vi "UpdateChannelWithParams.vi"(8 "error in":errorcluster, 10 "ParamArray":T1[](array[typedef]), 11 "channels in":T5 {"speed" items=["OWL429_HIGH_SPEED_CHANNEL", "OWL429_LOW_SPEED_CHANNEL"]; "Labels"."scheduleBuildUnit" items=["Millisecond", "Microsecond"]}) -> (0 "error out":errorcluster, 3 "channels out":T5 {"speed" items=["OWL429_HIGH_SPEED_CHANNEL", "OWL429_LOW_SPEED_CHANNEL"]; "Labels"."scheduleBuildUnit" items=["Millisecond", "Microsecond"]})   [LabVIEW 2016]
uses:
  Ballard Arinc-429 System Explorer.lvlib
  Controls/ARINCParam.ctl
  Controls/AIT_Label.ctl
  Controls/AIT_Channel.ctl
  Controls/AIT_Channel Array.ctl
  Controls/LabelInfo.ctl
  Controls/LabelParam.ctl
  Controls/ChannelParams.ctl
  Controls/AIT_Word.ctl
  Shared/Controls and Global/TransferType.ctl
  Shared/Ballard Arinc-429 Shared.lvlib
  Controls/Channel_direction.ctl
  Controls/Channel Speed.ctl
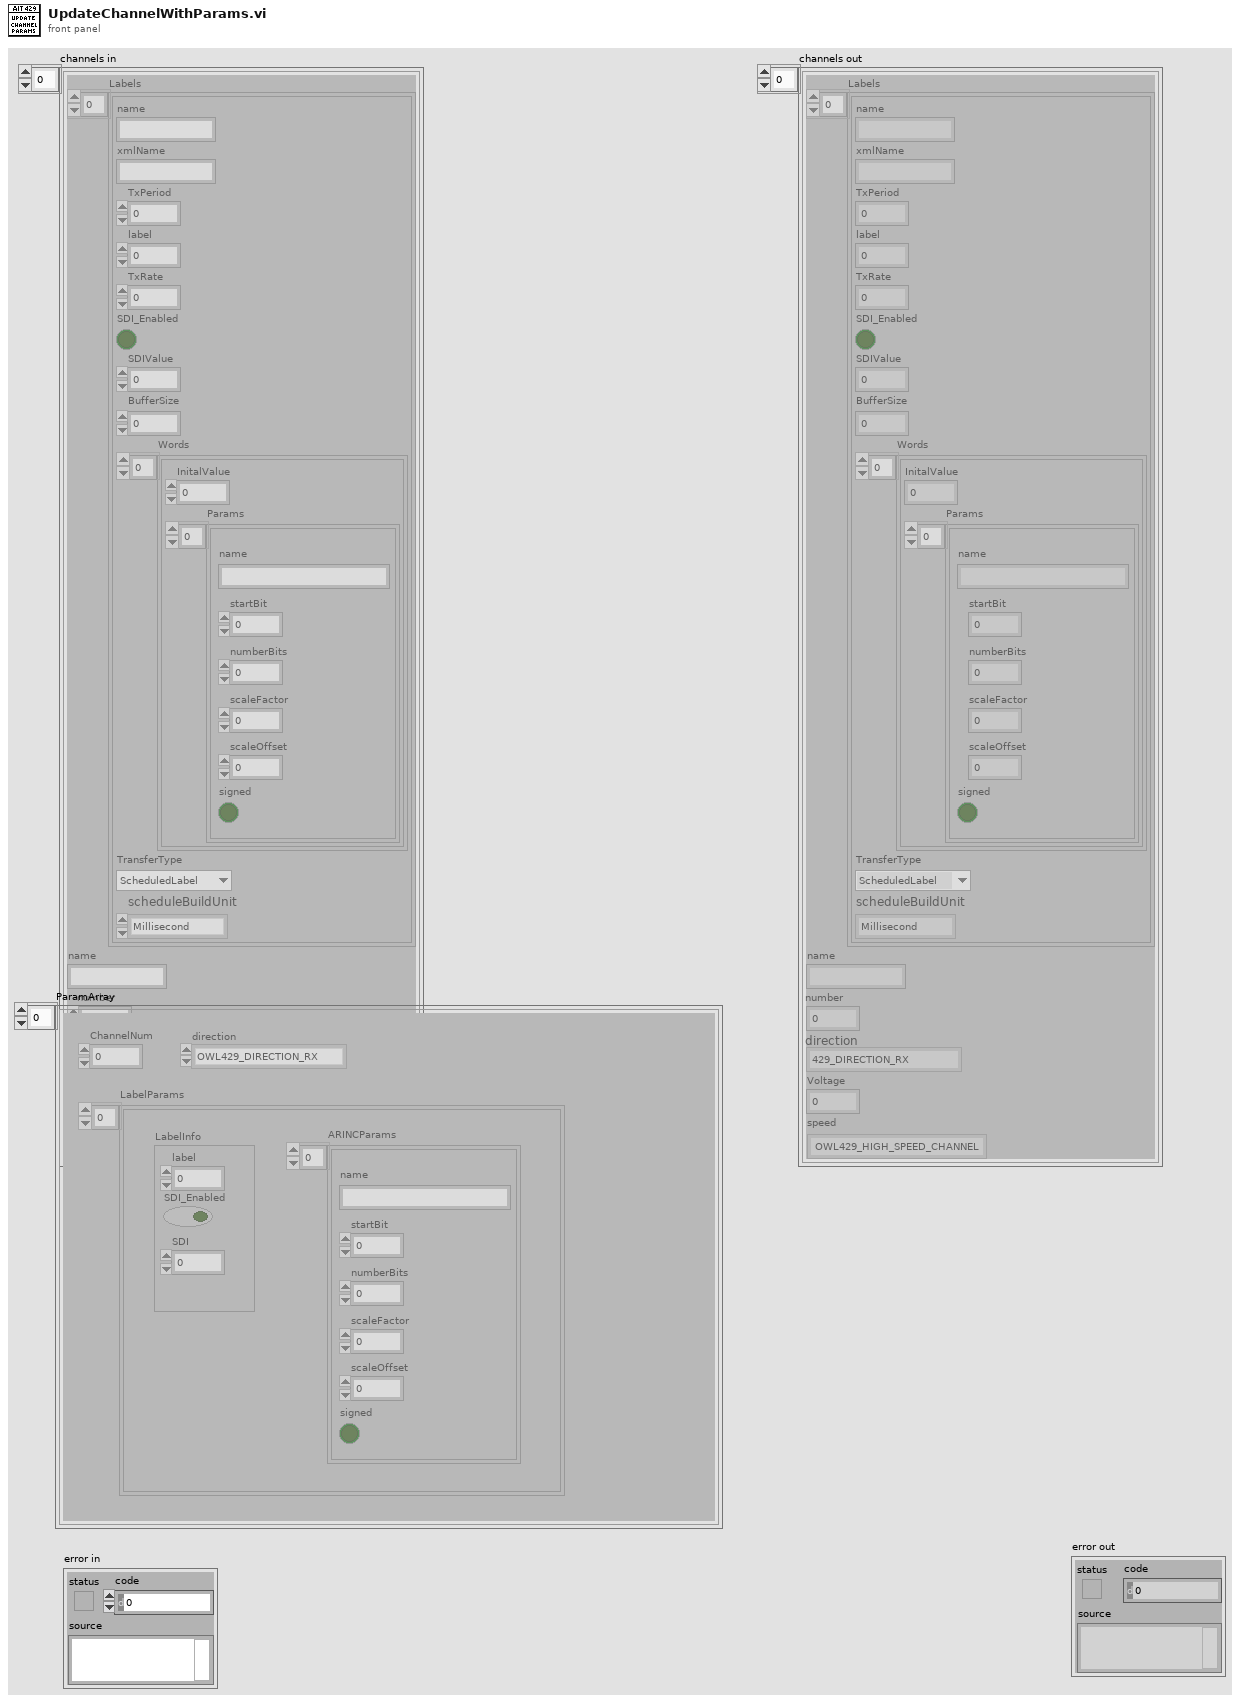
[diagram p1: front panel]
types:
  T1 = typedef "Ballard Arinc-429 System Explorer.lvlib/ChannelParams.ctl" = cluster{"ChannelNum":u8, "LabelParams":T2[], "direction":enum16{"OWL429_DIRECTION_RX", "OWL429_DIRECTION_TX"}}
  T2 = typedef "Ballard Arinc-429 System Explorer.lvlib/LabelParam.ctl" = cluster{"LabelInfo":T3, "ARINCParams":T4[]}
  T3 = typedef "Ballard Arinc-429 System Explorer.lvlib/LabelInfo.ctl" = cluster{"label":u32, "SDI_Enabled":bool, "SDI":u8}
  T4 = typedef "Ballard Arinc-429 System Explorer.lvlib/ARINCParam.ctl" = cluster{"name":string, "startBit":i32, "numberBits":i32, "scaleFactor":dbl, "scaleOffset":dbl, "signed":bool}
  T5 = typedef "Ballard Arinc-429 System Explorer.lvlib/AIT_Channel Array.ctl" = T6[]
  T6 = typedef "Ballard Arinc-429 System Explorer.lvlib/AIT_Channel.ctl" = cluster{"Labels":T7[], "name":string, "number":u8, "direction":T10, "Voltage":dbl, "speed":T11}
  T7 = typedef "Ballard Arinc-429 System Explorer.lvlib/AIT_Label.ctl" = cluster{"name":string, "xmlName":string, "TxPeriod":u32, "label":u32, "TxRate":dbl, "SDI_Enabled":bool, "SDIValue":u8, "BufferSize":u32, "Words":T8[], "TransferType":T9, "scheduleBuildUnit":i32}
  T8 = typedef "Ballard Arinc-429 System Explorer.lvlib/AIT_Word.ctl" = cluster{"InitalValue":u32, "Params":T4[]}
  T9 = typedef "Ballard Arinc-429 Shared.lvlib/TransferType.ctl" = enum16{"ScheduledLabel", "Acyclic", "Block", "Strobe"}
  T10 = typedef "Channel_direction.ctl" = enum16{"429_DIRECTION_RX", "429_DIRECTION_TX"}
  T11 = typedef "Channel Speed.ctl" = i32
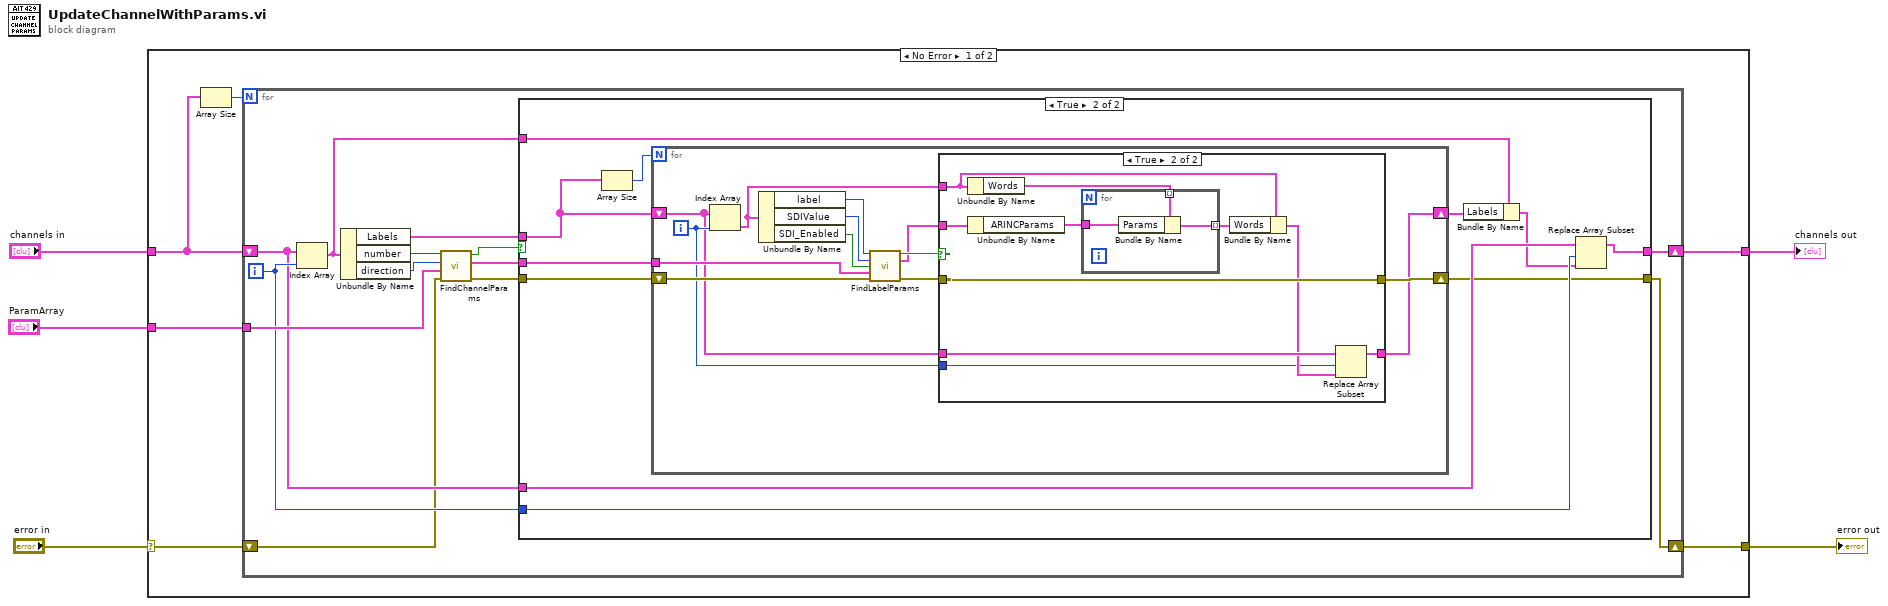
[diagram p0: block diagram]
diagram:
  n1 = case shown="No Error" "error in" {
    selector: "error in" -> [w7 w67]
    tunnel: [w11 w66] -> w5
    tunnel: "channels in" -> [w10 w66]
    tunnel: "ParamArray" -> [w8 _]
    tunnel: [w6 w67] -> w1
    frame No Error {
      n2 = Array Size(array=w10) -> (size(s)=w9:i32)
      n3 = for {
        N: w9 -> [_]
        tunnel: w8 -> [w22]
        shift-right: [w14] -> w11
        shift-left: w10 -> [w16]
        shift-right: [w12] -> w6
        shift-left: w7 -> [w13]
        i -> [w17]
        n4 = Index Array(array=w16, index=w17) -> (element=w15:T6)
        n5 = Unbundle By Name(w15) -> ("Labels"=w18:T7[], "number"=w24:u8, "direction"=w23:T10)
        n6 = call "FindChannelParams.vi"("error in"=w13, "ChannelParams"=w22, "Direction"=w23, "ChannelNumber"=w24) -> ("error out"=w21:errorcluster, "LabelParams"=w19:T2[], "Found"=w20:bool)  [unwired: 5 in]
        n7 = case shown="True" w20 {
          tunnel: w21 -> [w25 w37]
          tunnel: w19 -> [_ w36]
          tunnel: w18 -> [_ w34]
          tunnel: w17 -> [_ w32]
          tunnel: w16 -> [w26 w33]
          tunnel: w15 -> [_ w31]
          tunnel: [w26 w28] -> w14
          tunnel: [w25 w27] -> w12
          frame False {
          }
          frame True {
            n8 = Array Size(array=w34) -> (size(s)=w35:i32)
            n9 = for {
              N: w35 -> [_]
              shift-right: [w43] -> w27
              shift-left: w37 -> [w50]
              tunnel: w36 -> [w47]
              shift-right: [w39] -> w30
              shift-left: w34 -> [w40]
              i -> [w41]
              n10 = Index Array(array=w40, index=w41) -> (element=w42:T7)
              n11 = Unbundle By Name(w42) -> ("label"=w38:u32, "SDIValue"=w49:u8, "SDI_Enabled"=w48:bool)
              n12 = call "FindLabelParams.vi"("label"=w38, "SDI"=w49, "SDI_Enabled"=w48, "LabelParamsArray"=w47, "error in"=w50) -> ("Found"=w46:bool, "LabelParams"=w44:T2, "error out"=w45:errorcluster)  [unwired: 8 in]
              n13 = case shown="True" w46 {
                tunnel: w45 -> [w52 w61]
                tunnel: w44 -> [_ w62]
                tunnel: [w52 w61] -> w43
                tunnel: w42 -> [_ w54]
                tunnel: w41 -> [_ w53]
                tunnel: w40 -> [w51 w60]
                tunnel: [w51 w59] -> w39
                frame False {
                }
                frame True {
                  n14 = Unbundle By Name(w54) -> ("Words"=w58:T8[])
                  n15 = Unbundle By Name(w62) -> ("ARINCParams"=w57:T4[])
                  n16 = for {
                    tunnel: w58 -> [w65] mode=indexing
                    tunnel: w57 -> [w64]
                    tunnel: [w63] -> w56 mode=indexing
                    n17 = Bundle By Name(cluster=w65, "Params"=w64) -> (w63:T8)
                  }
                  n18 = Bundle By Name(cluster=w54, "Words"=w56) -> (w55:T7)
                  n19 = Replace Array Subset(array=w60, new element=w55, index=w53) -> (w59:T7[])
                }
              }
            }
            n20 = Bundle By Name(cluster=w31, "Labels"=w30) -> (w29:T6)
            n21 = Replace Array Subset(array=w33, new element=w29, index=w32) -> (w28:T5)
          }
        }
      }
    }
    frame Error {
    }
  }
  "channels out" <- w5
  "error out" <- w1
